vi "test_MonoSlitInMM.vi"(8 "error in":errorcluster, 11 "Monochromator in":refnum<class "Monochromator.lvclass">) -> (0 "error out":errorcluster, 3 "Monochromator out":refnum<class "Monochromator.lvclass">)   [LabVIEW 2020, in "horiba.test.lvlib"]
uses:
  horiba.test.lvlib
  Classes/Mono/Monochromator.lvclass
  <vilib>/addons/_JKI Toolkits/Caraya/classes/Assert/Assert Almost Equal_Float.vi
panel:
  # "Connector Pane"
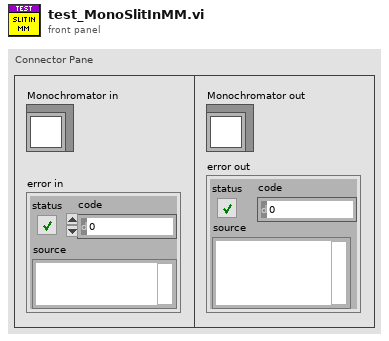
[diagram p1: front panel]
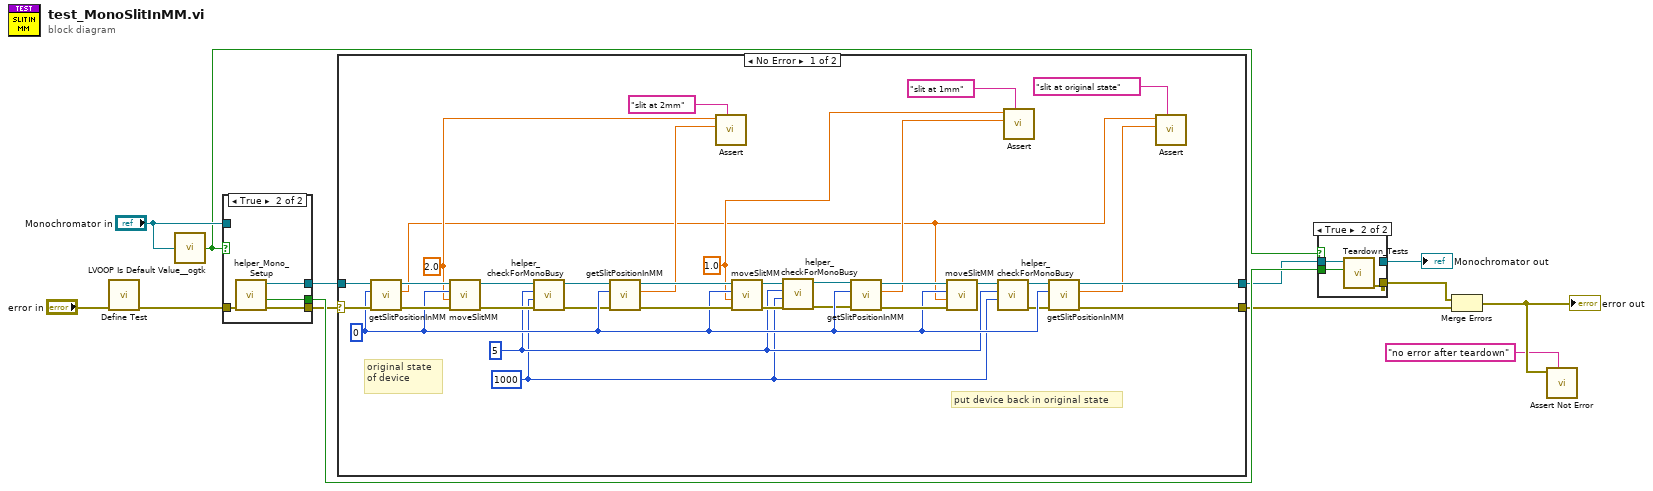
[diagram p0: block diagram]
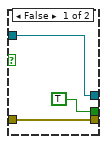
[diagram p2: hidden frame]
diagram:
  n1 = call <vilib>:"Define Test.vi"("error in (no error)"="error in") -> ("error out"=w7:errorcluster)  [unwired: 9 in, 1 out]
  n2 = call <userlib>:"LVOOP Is Default Value__ogtk.vi"("Object"="Monochromator in") -> ("Is Default Value?"=w8:bool)
  n3 = case shown="True" w8 {
    tunnel: w7 -> [w15 w20]
    tunnel: [w15 w19] -> w2
    tunnel: [w16 w18] -> w5
    tunnel: [TRUE ("Module Was Already Running?") w17] -> w10
    tunnel: "Monochromator in" -> [w16 _]
    frame False {
    }
    frame True {
      n4 = call "helper_Mono_Setup.vi"("error in"=w20) -> ("error out"=w19:errorcluster, "Module Was Already Running?"=w17:bool, "Monochromator out"=w18:refnum<class "Monochromator.lvclass">)  [unwired: 7 in, 1 out]
    }
  }
  n5 = case shown="No Error" w2 {
    selector: w2 -> [w46 w55]
    tunnel: [w37 w54] -> w4
    tunnel: w5 -> [w45 w54]
    tunnel: [w36 w55] -> w1
    frame No Error {
      w21 = u32 1000 ("milliseconds to wait")
      w22 = 5
      w44 = 0 ("locationId")
      w39 = 1.0 ("position")
      w43 = 2.0 ("position")
      # "put device back in original state"
      # "original state of device"
      n6 = call "getSlitPositionInMM.vi"("error in (no error)"=w46, "locationId"=w44, "Monochromator in"=w45) -> ("error out"=w51:errorcluster, "position"=w34:dbl, "Monochromator out"=w52:refnum<class "Monochromator.lvclass">)  [unwired: 6 in]
      n7 = call "moveSlitMM.vi"("error in (no error)"=w51, "position"=w43, "locationId"=w44, "Monochromator in"=w52) -> ("error out"=w32:errorcluster, "Monochromator out"=w33:refnum<class "Monochromator.lvclass">)  [unwired: 4 in, 2 out]
      n8 = call "helper_checkForMonoBusy.vi"("error in (no error)"=w32, "milliseconds to wait"=w21, "Numeric"=w22, "Monochromator in"=w33) -> ("error out"=w30:errorcluster, "Monochromator out"=w31:refnum<class "Monochromator.lvclass">)  [unwired: 5 in, 1 out]
      n9 = call "getSlitPositionInMM.vi"("error in (no error)"=w30, "locationId"=w44, "Monochromator in"=w31) -> ("error out"=w49:errorcluster, "position"=w42:dbl, "Monochromator out"=w50:refnum<class "Monochromator.lvclass">)  [unwired: 6 in]
      n10 = call-poly <vilib>:"Assert.vi"("Label"="slit at 2mm", "Y"=w42, "X"=w43) -> ()  [unwired: 7 in, 2 out]
      n11 = call "moveSlitMM.vi"("error in (no error)"=w49, "position"=w39, "locationId"=w44, "Monochromator in"=w50) -> ("error out"=w29:errorcluster, "Monochromator out"=w28:refnum<class "Monochromator.lvclass">)  [unwired: 4 in, 2 out]
      n12 = call "helper_checkForMonoBusy.vi"("error in (no error)"=w29, "milliseconds to wait"=w21, "Numeric"=w22, "Monochromator in"=w28) -> ("error out"=w27:errorcluster, "Monochromator out"=w26:refnum<class "Monochromator.lvclass">)  [unwired: 5 in, 1 out]
      n13 = call "getSlitPositionInMM.vi"("error in (no error)"=w27, "locationId"=w44, "Monochromator in"=w26) -> ("error out"=w47:errorcluster, "position"=w40:dbl, "Monochromator out"=w48:refnum<class "Monochromator.lvclass">)  [unwired: 6 in]
      n14 = call "moveSlitMM.vi"("error in (no error)"=w47, "position"=w34, "locationId"=w44, "Monochromator in"=w48) -> ("Monochromator out"=w23:refnum<class "Monochromator.lvclass">)  [unwired: 4 in, 3 out]
      n15 = call "helper_checkForMonoBusy.vi"("milliseconds to wait"=w21, "Numeric"=w22, "Monochromator in"=w23) -> ("error out"=w25:errorcluster, "Monochromator out"=w24:refnum<class "Monochromator.lvclass">)  [unwired: 6 in, 1 out]
      n16 = call-poly <vilib>:"Assert.vi"("Label"="slit at 1mm", "Y"=w40, "X"=w39) -> ()  [unwired: 7 in, 2 out]
      n17 = call "getSlitPositionInMM.vi"("error in (no error)"=w25, "locationId"=w44, "Monochromator in"=w24) -> ("error out"=w36:errorcluster, "position"=w35:dbl, "Monochromator out"=w37:refnum<class "Monochromator.lvclass">)  [unwired: 6 in]
      n18 = call-poly <vilib>:"Assert.vi"("Label"="slit at original state", "Y"=w35, "X"=w34) -> ()  [unwired: 7 in, 2 out]
    }
    frame Error {
    }
  }
  n19 = case shown="True" w8 {
    tunnel: w4 -> [w56 w59]
    tunnel: [_ w58] -> w6
    tunnel: w10 -> [_ w57]
    tunnel: [w56 _] -> w3
    frame False {
    }
    frame True {
      n20 = call "Teardown_Tests.vi"("Module Was Already Running?"=w57, "horiba.lvlib:GenericDevice"=w59) -> ("error out"=w58:errorcluster)  [unwired: 8 in, 1 out]
    }
  }
  "Monochromator out" <- w3
  n21 = Merge Errors(w6, w1) -> (w12:errorcluster)
  "error out" <- w12
  n22 = call <vilib>:"Assert Not Error.vi"("Label"="no error after teardown", "Not Error?"=w12) -> ()  [unwired: 8 in, 2 out]
